vi "Configure Programmer Parameters.vi"(0 "VISA resource name":refnum<visa-resource-name>, 1 "Unit Address (1)":u8=1 min=1 max=254, 5 "Program Cycles (1)":i16=1, 7 "Segment Weighting":bool[](array[boolean]), 9 "Event Output (False: Disable)":bool, 11 "error in (no error)":errorcluster) -> (4 "VISA resource name out":refnum<visa-resource-name>, 15 "error out":errorcluster)   [LabVIEW 2010, in "Eurotherm 32xx Series.lvlib"]
doc: "This VI sets Programmer/Timer parameters."
uses:
  <instrlib>/Eurotherm 32xx Series/Eurotherm 32xx Series.lvlib
panel:
  # "Ramp 1"
  # "Dwell 1"
  # "Ramp 2"
  # "Dwell 2"
  # "Ramp 3"
  # "Dwell 3"
  # "Ramp 4"
  # "Ramp 4"
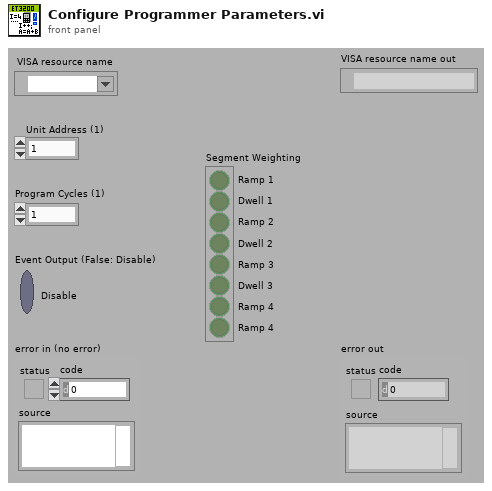
[diagram p1: front panel]
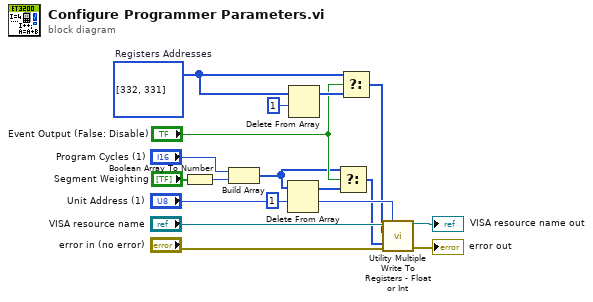
[diagram p0: block diagram]
diagram:
  w6 = u16[] [332, 331]  # Registers Addresses
  n1 = Boolean Array To Number(Boolean array="Segment Weighting") -> (number=w1:u32)
  n2 = Build Array("Program Cycles (1)", w1) -> (w3:u32[])
  n3 = Delete From Array(array=w3, length=1) -> (array with subset deleted=w8:u32[])  [unwired: 1 in, 1 out]
  n4 = Delete From Array(array=w6, length=1) -> (array with subset deleted=w7:u16[])  [unwired: 1 in, 1 out]
  n5 = Select(t=w3, s="Event Output (False: Disable)", f=w8) -> (s? t:f=w2:u32[])
  n6 = Select(t=w6, s="Event Output (False: Disable)", f=w7) -> (s? t:f=w5:u16[])
  n7 = call <instrlib>:"Utility Multiple Write To Registers - Float or Int.vi"("VISA resource name"="VISA resource name", "Unit Address (1)"="Unit Address (1)", "Registers Addresses (0)"=w5, "Data (0)"=w2, "error in (no error)"="error in (no error)") -> ("VISA resource name out"=→"VISA resource name out":refnum<visa-resource-name>, "error out"=→"error out":errorcluster)  [unwired: 9 in]
